vi "axisSpan.vi"(10 "DataSpan":cluster{"Max":dbl, "Min":dbl}, 11 "AxisBounds":T1) -> (3 "ActualSpan":dbl)   [LabVIEW 2013]
uses:
  minAndMax.ctl
  AutoManualNumber.ctl
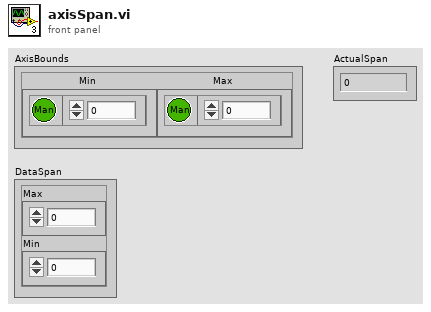
[diagram p1: front panel]
types:
  T1 = typedef "minAndMax.ctl" = cluster{"Min":T2, "Max":T2}
  T2 = typedef "AutoManualNumber.ctl" = cluster{"Auto":bool, "Value":dbl}
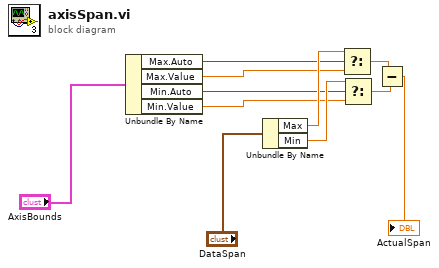
[diagram p0: block diagram]
diagram:
  n1 = Unbundle By Name("AxisBounds") -> ("Max.Auto"=w1:bool, "Max.Value"=w2:dbl, "Min.Auto"=w3:bool, "Min.Value"=w4:dbl)
  n2 = Unbundle By Name("DataSpan") -> ("Max"=w10:dbl, "Min"=w11:dbl)
  n3 = Select(t=w10, s=w1, f=w2) -> (s? t:f=w6:dbl)
  n4 = Select(t=w11, s=w3, f=w4) -> (s? t:f=w7:dbl)
  n5 = Subtract(x=w6, y=w7) -> (x-y=→"ActualSpan":dbl)
